vi "Simulated Console.vi"(8 "error in (no error)":errorcluster, 9 "Module Routes":refnum<user-event>[](array[refnum]), 11 "Event Registration Refnum":refnum<event-registration>) -> (0 "error out":errorcluster)   [LabVIEW 2018]
doc: "Simulated console UI"
uses:
  Architecture/Message Queue/Message Cluster.ctl
  Controls/Console Status.ctl
  Controls/Entry Display.ctl
  Car Wash Controller/Controls/Steps.ctl
  Car Wash Controller/Controls/Stations.ctl
  Architecture/Modules.ctl
  Controls/Button state.ctl
  Architecture/Message Queue/Message Queue.lvlib
panel:
  in  "Vehicle Position Simulation":u32(slide) scale=0.0..4.0
  out "Time Remaining":dbl format="%6.2f Seconds"
  out "Out of Position?":bool caption="Vehicle out of position"
  out "Air Dry":bool
  out "Tire Shine Foam":bool
  out "Spot Free Rinse":bool
  out "Low Pressure Wax":bool
  out "High Pressure Wash":bool
  out "Pre-Soak":bool
  out "Bug Remover":bool
  out "Under Body Wash":bool
  out "Wash Entry":string
  in  "Wash Start":bool
  in  "Air Dry":bool
  in  "Tire Shine Foam":bool
  in  "Spot Free Rinse":bool
  in  "Low Pressure Wax":bool
  in  "High Pressure Wash (default)":bool
  in  "Pre-Soak":bool
  in  "Bug Remover":bool
  in  "Under Body Wash":bool
  in  "debug":bool
  # "[Covers: UI2]\n[Covers UI2A]"
  # "[Covers: UI3]\n[Covers: UI3A]"
  # "[Covers: UI1]"
  # "Entry Console"
  # "Wash Display Console"
  # "[Covers: UI3B]\n[Covers: UI3B1]"
  # "[Covers: UI2B]"
  # "[Covers: UI3C]\n[Covers: UI3C1]\n[Covers: UI3C2]"
  # "[Covers: UI3D]\n[Covers: UI3D1]"
  # "Vehicle Position Simulation"
  # "[Covers: UI4]\n[Covers: UI4A]"
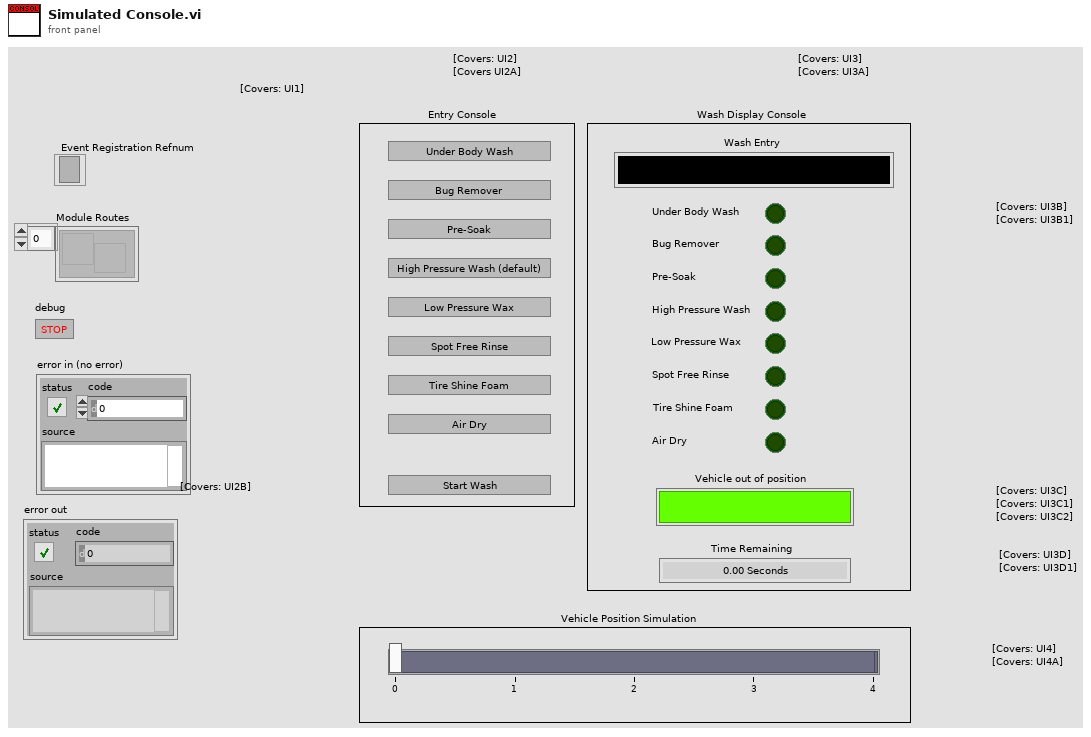
[diagram p1: front panel]
types:
  T1 = typedef "Console Status.ctl" = cluster{"Module Routes":refnum<user-event>[], "Chosen Cycles":cluster{"Under Body Wash":bool, "Bug Remover":bool, "Pre-Soak":bool, "High Pressure Wash (default)":bool, "Low Pressure Wax":bool, "Spot Free Rinse":bool, "Tire Shine Foam":bool, "Air Dry":bool}, "Entry Display":T2, "Current State":T3, "In Progress?":bool, "Out of Position?":bool, "Time Remaining":dbl, "Current Station":T4}
  T2 = typedef "Entry Display.ctl" = cluster{"Text":string, "Color":u32}
  T3 = typedef "Steps.ctl" = enum16{"Under Body Wash", "Bug Remover", "Pre-Soak", "High Pressure Wash", "Low Pressure Wax", "Spot Free Rinse", "Tire Shine Foam", "Air Dry"}
  T4 = typedef "Stations.ctl" = enum16{"Entry", "Station 1", "Station 2", "Station 3", "Exit"}
  T5 = typedef "Modules.ctl" = enum16{"Database", "Car Wash Controller", "Console"}
  T6 = typedef "Button state.ctl" = cluster{"Disabled State":enum8{"Enabled", "Disabled", "Disabled and Grayed Out"}, "State":bool}
  T7 = cluster{"[0]":bool, "[1]":bool, "[2]":bool, "[3]":bool, "[4]":bool, "[5]":bool, "[6]":bool, "[7]":bool}
  T8 = typedef "Error Severity.ctl" = enum16{"System Error", "Wash Error", "Minor"}
  T9 = cluster{"Under Body Wash":bool, "Bug Remover":bool, "Pre-Soak":bool, "High Pressure Wash (default)":bool, "Low Pressure Wax":bool, "Spot Free Rinse":bool, "Tire Shine Foam":bool, "Air Dry":bool}
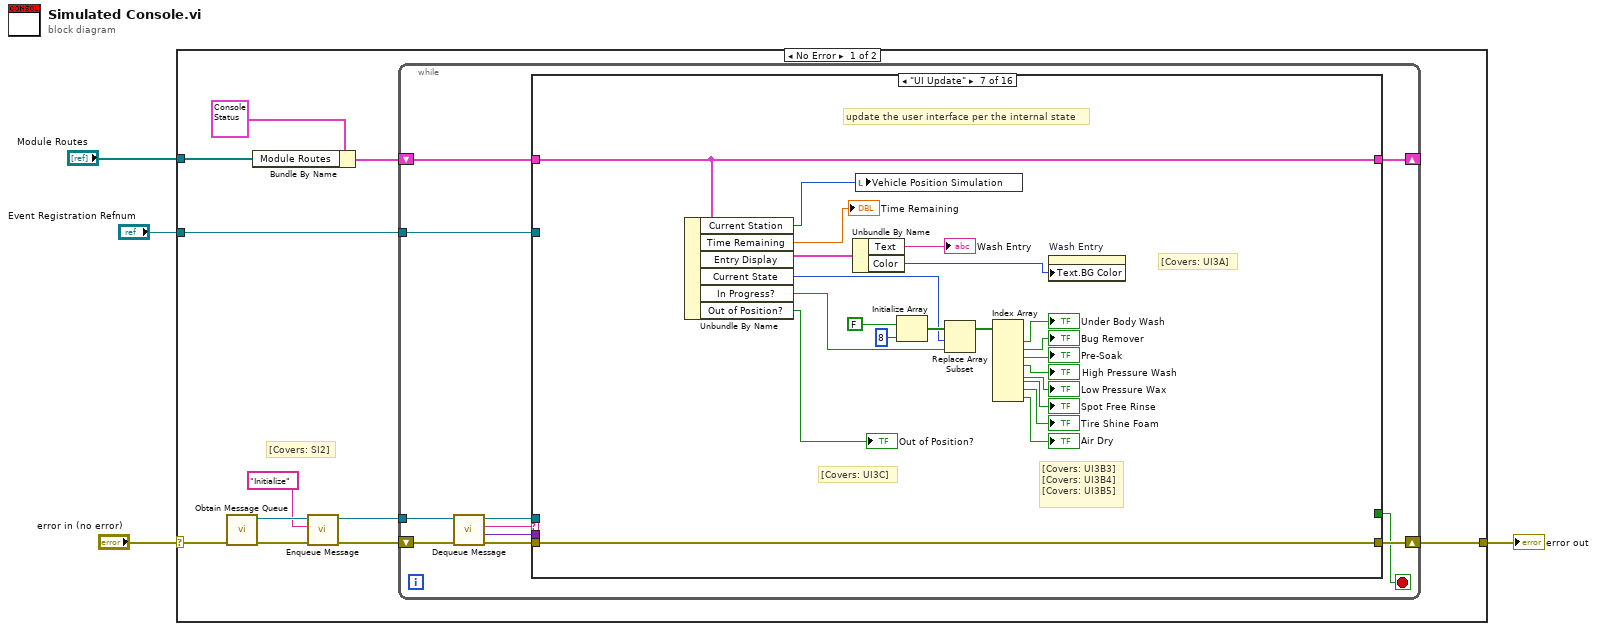
[diagram p0: block diagram]
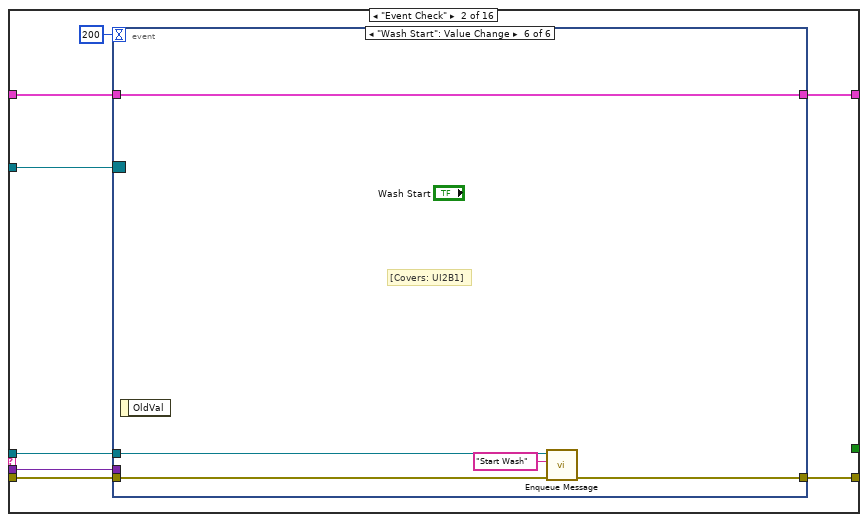
[diagram p3: hidden frame]
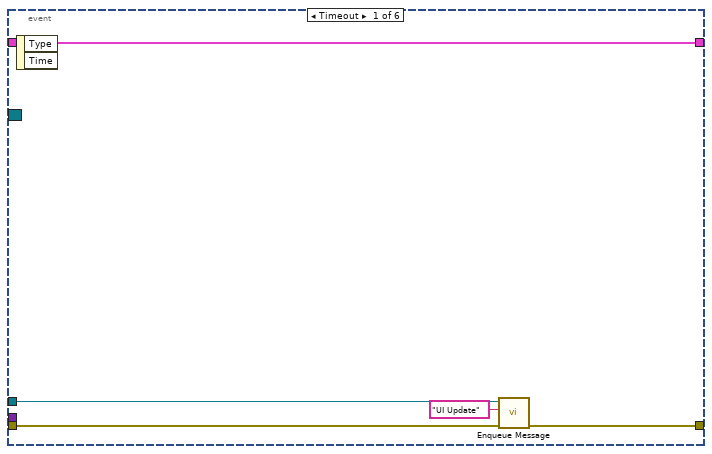
[diagram p4: hidden frame]
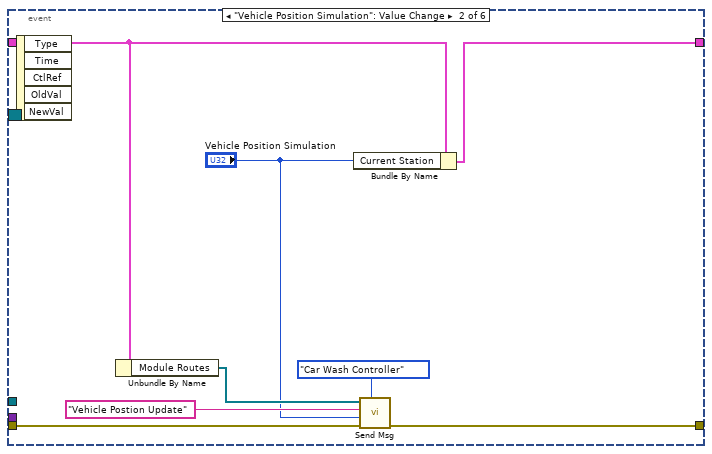
[diagram p5: hidden frame]
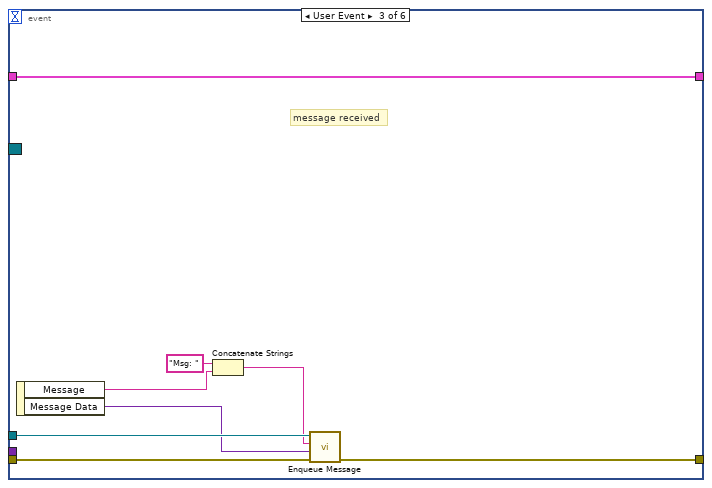
[diagram p6: hidden frame]
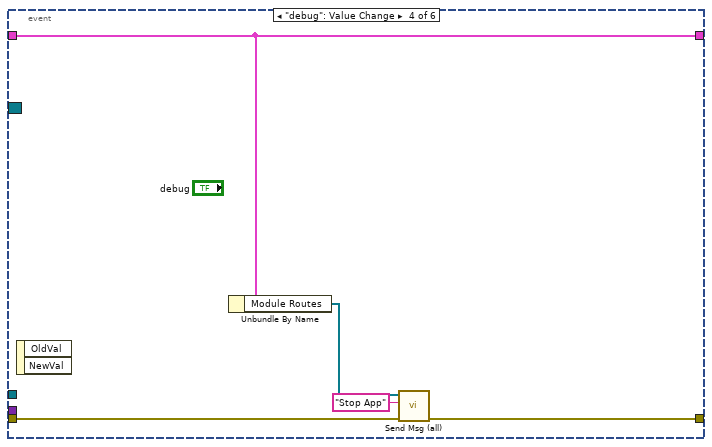
[diagram p7: hidden frame]
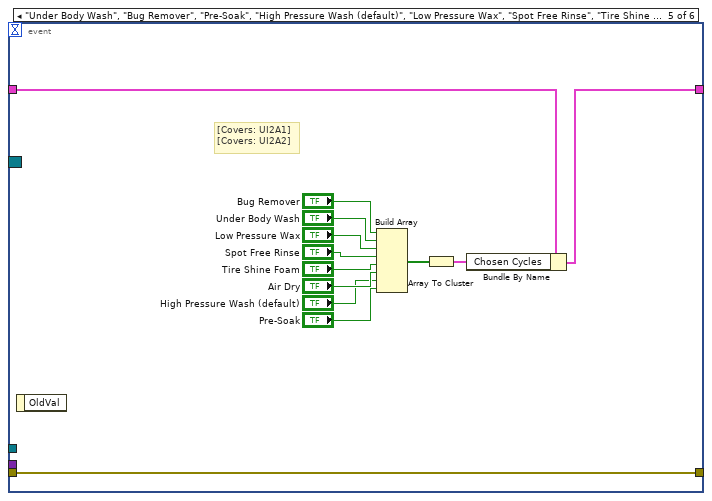
[diagram p8: hidden frame]
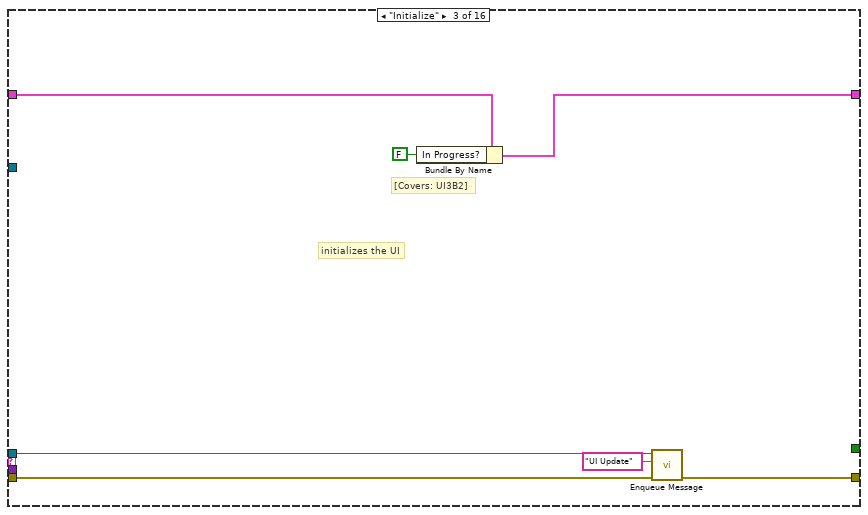
[diagram p9: hidden frame]
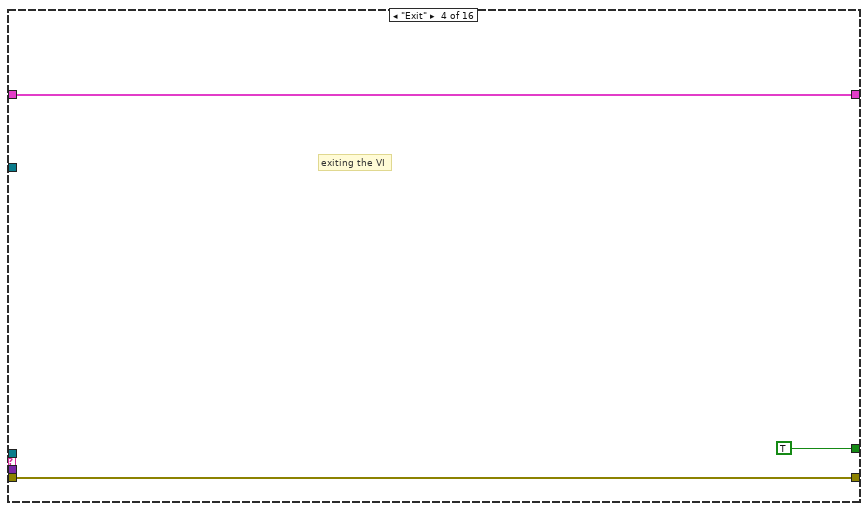
[diagram p10: hidden frame]
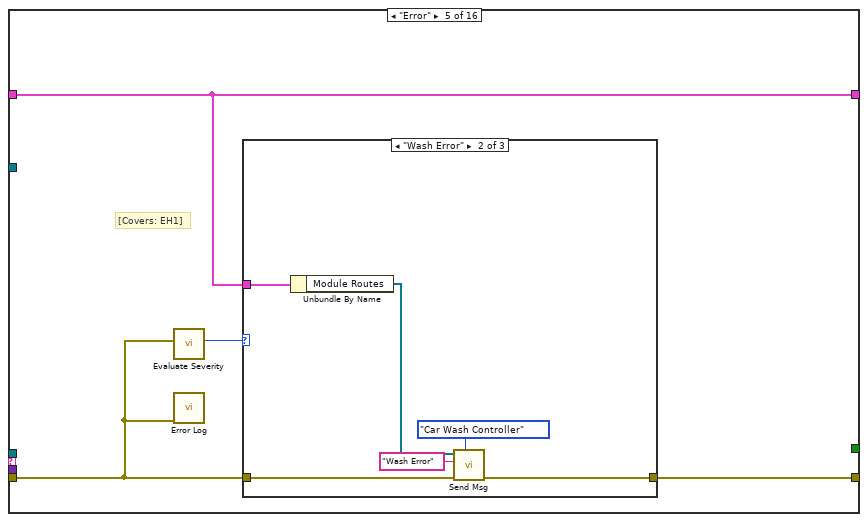
[diagram p11: hidden frame]
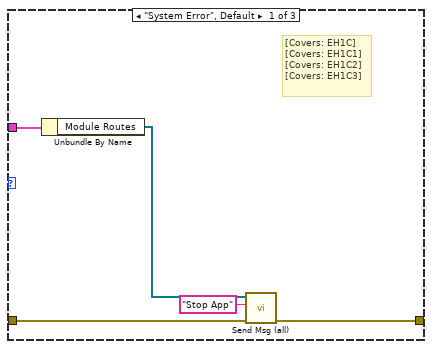
[diagram p12: hidden frame]
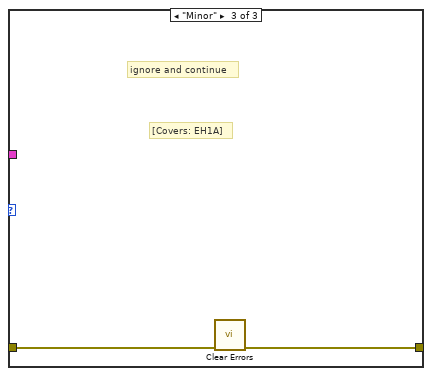
[diagram p13: hidden frame]
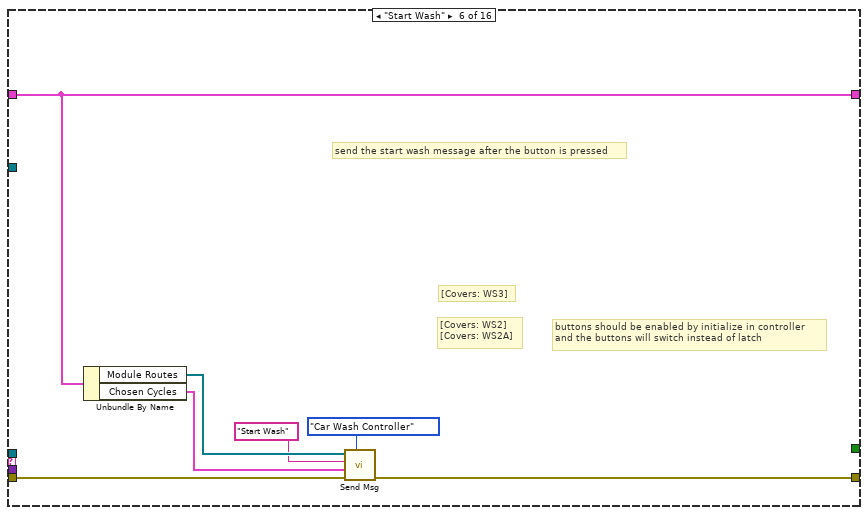
[diagram p14: hidden frame]
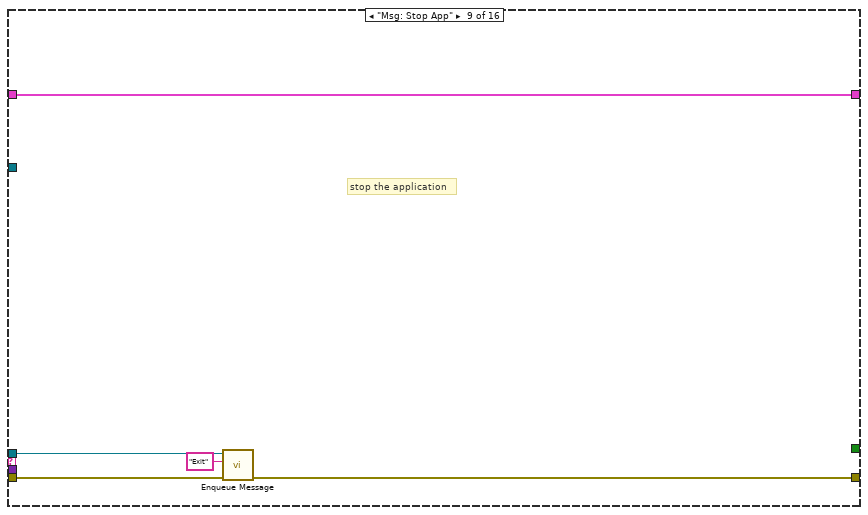
[diagram p16: hidden frame]
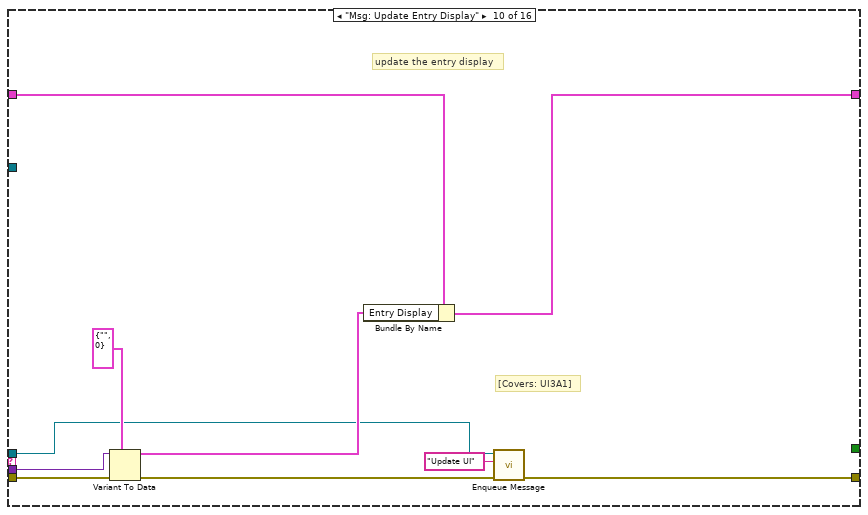
[diagram p17: hidden frame]
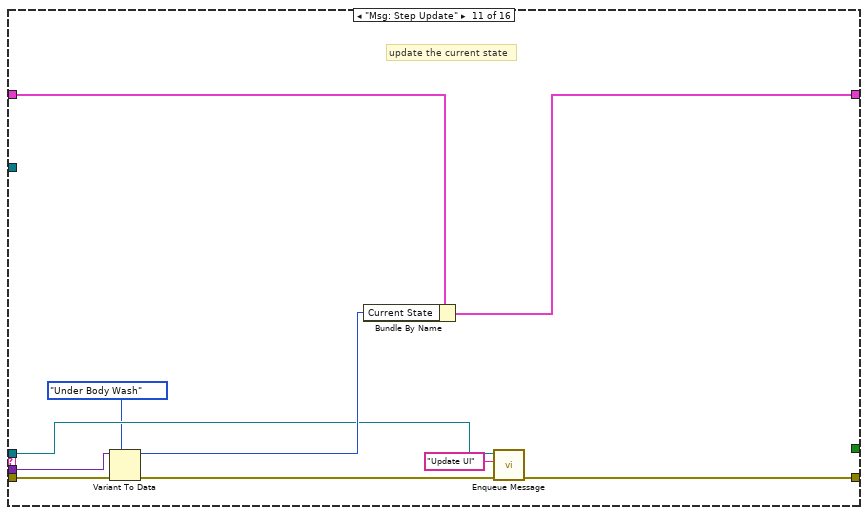
[diagram p18: hidden frame]
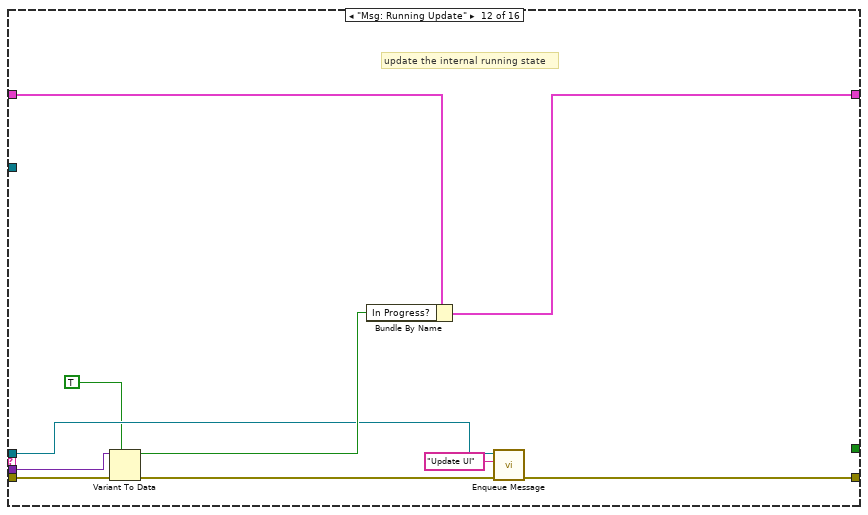
[diagram p19: hidden frame]
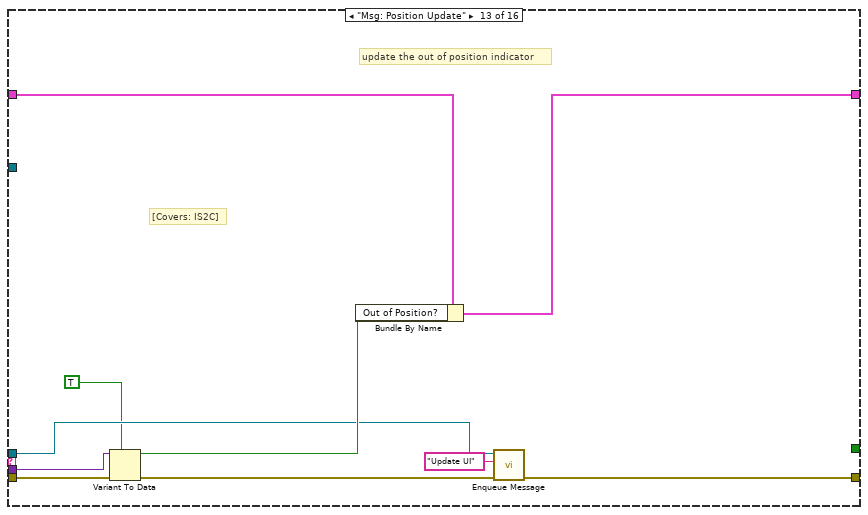
[diagram p20: hidden frame]
diagram:
  n1 = case shown="No Error" "error in (no error)" {
    selector: "error in (no error)" -> [w12 w220]
    tunnel: "Module Routes" -> [w14 _]
    tunnel: "Event Registration Refnum" -> [w13 _]
    tunnel: [w6 w220] -> w1
    frame No Error {
      # "[Covers: SI2]"
      n2 = call "Obtain Message Queue.vi"("error in (no error)"=w12) -> ("error out"=w11:errorcluster, "Message Queue"=w10:refnum<queue>)  [unwired: 9 in]
      n3 = Bundle By Name(cluster=T1 {"Module Routes"=[], "Chosen Cycles"={"Under Body Wash"=FALSE, "Bug Remover"=FALSE, "Pre-Soak"=FALSE, "High Pressure Wash (default)"=FALSE, "Low Pressure Wax"=FALSE, "Spot Free Rinse"=FALSE, "Tire Shine Foam"=FALSE, "Air Dry"=FALSE}, "Entry Display"={"Text"="", "Color"=0}, "Current State"=enum."Under Body Wash", "In Progress?"=FALSE, "Out of Position?"=FALSE, "Time Remaining"=0.0, "Current Station"=enum."Entry"} ("Status"), "Module Routes"=w14) -> (w5:T1)
      n4 = call "Enqueue Message.vi"("error in (no error)"=w11, "Message"="Initialize", "Message Queue"=w10) -> ("error out"=w8:errorcluster, "dup Message Queue"=w7:refnum<queue>)  [unwired: 7 in]
      n5 = while {
        tunnel: w13 -> [w26]
        shift-right: [w22] -> w6
        shift-left: w8 -> [w25]
        tunnel: w7 -> [w24]
        shift-right: [w16] -> _
        shift-left: w5 -> [w17]
        stop <- w18 stop-if-true
        n6 = call "Dequeue Message.vi"("error in (no error)"=w25, "Message Queue"=w24) -> ("error out"=w23:errorcluster, "Message Data"=w20:variant, "Message"=w19:string, "dup Message Queue"=w21:refnum<queue>)  [unwired: 6 in]
        n7 = case shown="\"UI Update\"" w19 {
          tunnel: w26 -> [_ w36 _ _ _ _ _ _ _ _ _ _ _ _ _ _]
          tunnel: w23 -> [w28 w35 w84 w90 w91 w114 w136 w138 w142 w153 w163 w173 w183 w193 w203 w219]
          tunnel: [w28 w34 w82 w90 w93 w113 w136 w138 w140 w144 w155 w165 w175 w185 w196 w216] -> w22
          tunnel: w21 -> [_ w33 w83 _ _ _ _ _ w141 w146 w157 w167 w177 w187 w198 _]
          tunnel: w20 -> [_ w32 _ _ _ _ _ _ _ w151 w162 w172 w182 w192 w202 w218]
          tunnel: [_ _ _ TRUE _ _ _ _ _ _ _ _ _ _ _ _] -> w18
          tunnel: w17 -> [w27 w31 w87 w88 w92 w112 w135 w137 w143 w150 w161 w171 w181 w191 w201 w215]
          tunnel: [w27 w30 w86 w88 w92 w112 w135 w137 w143 w149 w160 w170 w180 w190 w200 w215] -> w16
          frame Default {
            # "invalid case"
          }
          frame "Event Check" {
            n8 = event shown="[5] \"Wash Start\": Value Change" {
              selector: w36 -> [_ _ _ _ _ _]
              dyn-events: _ -> [_ _ _ _ _ _]
              timeout: 200 -> [_ _ _ _ _ _]
              tunnel: [w39 w47 w54 w61 w75 w78] -> w34
              tunnel: w35 -> [w40 w48 w55 w62 w75 w79]
              tunnel: w33 -> [w38 _ w53 _ _ w77]
              tunnel: w32 -> [_ _ _ _ _ _]
              tunnel: w31 -> [w41 w45 w50 w60 w65 w80]
              tunnel: [w41 w49 w50 w60 w64 w80] -> w30
              event Timeout {
                n9 = event-data() -> ()  [unwired: 1 in, 2 out]
                n10 = call "Enqueue Message.vi"("error in (no error)"=w40, "Message"="UI Update", "Message Queue"=w38) -> ("error out"=w39:errorcluster)  [unwired: 7 in, 1 out]
              }
              event "Vehicle Position Simulation": Value Change {
                n11 = event-data() -> ()  [unwired: 1 in, 5 out]
                n12 = Unbundle By Name(w45) -> ("Module Routes"=w44:refnum<user-event>[])
                n13 = Bundle By Name(cluster=w45, "Current Station"="Vehicle Position Simulation") -> (w49:T1)
                n14 = call "Send Msg.vi"("Module"=Modules."Car Wash Controller", "error in (no error)"=w48, "Message Data"="Vehicle Position Simulation", "Message"="Vehicle Postion Update", "Module Routes"=w44) -> ("error out"=w47:errorcluster)  [unwired: 6 in]
              }
              event User Event {
                # "message received"
                n15 = event-data() -> ("Message"=w56:string, "Message Data"=w52:variant)  [unwired: 1 in]
                n16 = Concatenate Strings("Msg: " ("string"), w56) -> (w51:string)
                n17 = call "Enqueue Message.vi"("error in (no error)"=w55, "Message Data"=w52, "Message"=w51, "Message Queue"=w53) -> ("error out"=w54:errorcluster)  [unwired: 6 in, 1 out]
              }
              event "debug": Value Change {
                n18 = event-data() -> ()  [unwired: 1 in, 2 out]
                n19 = Unbundle By Name(w60) -> ("Module Routes"=w59:refnum<user-event>[])
                n20 = call "Send Msg (all).vi"("error in (no error)"=w62, "Message"="Stop App", "Module Routes"=w59) -> ("error out"=w61:errorcluster)  [unwired: 8 in]
              }
              event "Under Body Wash", "Bug Remover", "Pre-Soak", "High Pressure Wash (default)", "Low Pressure Wax", "Spot Free Rinse", "Tire Shine Foam", "Air Dry": Value Change {
                # "[Covers: UI2A1]\n[Covers: UI2A2]"
                n21 = event-data() -> ()  [unwired: 1 in, 1 out]
                n22 = Build Array("Bug Remover", "Under Body Wash", "Low Pressure Wax", "Spot Free Rinse", "Tire Shine Foam", "Air Dry", "High Pressure Wash (default)", "Pre-Soak") -> (w66:bool[])
                n23 = Array To Cluster(array=w66) -> (cluster=w63:T7)
                n24 = Bundle By Name(cluster=w65, "Chosen Cycles"=w63) -> (w64:T1)
              }
              event "Wash Start": Value Change {
                # "[Covers: UI2B1]"
                n25 = event-data() -> ()  [unwired: 1 in, 1 out]
                n26 = call "Enqueue Message.vi"("error in (no error)"=w79, "Message"="Start Wash", "Message Queue"=w77) -> ("error out"=w78:errorcluster)  [unwired: 7 in, 1 out]
              }
            }
          }
          frame "Initialize" {
            # "initializes the UI"
            # "[Covers: UI3B2]"
            n27 = Bundle By Name(cluster=w87, "In Progress?"=FALSE) -> (w86:T1)
            n28 = call "Enqueue Message.vi"("error in (no error)"=w84, "Message"="UI Update", "Message Queue"=w83) -> ("error out"=w82:errorcluster)  [unwired: 7 in, 1 out]
          }
          frame "Exit" {
            # "exiting the VI"
          }
          frame "Error" {
            # "[Covers: EH1]"
            n29 = call "Evaluate Severity.vi"("error in (no error)"=w91) -> ("Severity"=w94:T8)  [unwired: 10 in]
            n30 = call "Error Log.vi"("error in (no error)"=w91) -> ()  [unwired: 11 in]
            n31 = case shown="\"Wash Error\"" w94 {
              tunnel: w91 -> [w99 w104 w107]
              tunnel: [w98 w105 w106] -> w93
              tunnel: w92 -> [w97 w103 _]
              frame "System Error", Default {
                # "[Covers: EH1C]\n[Covers: EH1C1]\n[Covers: EH1C2]\n[Covers: EH1C3]"
                n32 = Unbundle By Name(w97) -> ("Module Routes"=w96:refnum<user-event>[])
                n33 = call "Send Msg (all).vi"("error in (no error)"=w99, "Message"="Stop App", "Module Routes"=w96) -> ("error out"=w98:errorcluster)  [unwired: 8 in]
              }
              frame "Wash Error" {
                n34 = Unbundle By Name(w103) -> ("Module Routes"=w102:refnum<user-event>[])
                n35 = call "Send Msg.vi"("Module"=Modules."Car Wash Controller", "error in (no error)"=w104, "Message"="Wash Error", "Module Routes"=w102) -> ("error out"=w105:errorcluster)  [unwired: 7 in]
              }
              frame "Minor" {
                # "[Covers: EH1A]"
                # "ignore and continue"
                n36 = call <vilib>:"Clear Errors.vi"("error in (no error)"=w107) -> ("error out"=w106:errorcluster)  [unwired: 5 in, 1 out]
              }
            }
          }
          frame "Start Wash" {
            # "send the start wash message after the button is pressed"
            # "buttons should be enabled by initialize in controller\nand the buttons will switch instead of latch"
            # "[Covers: WS2]\n[Covers: WS2A]"
            # "[Covers: WS3]"
            n37 = Unbundle By Name(w112) -> ("Module Routes"=w110:refnum<user-event>[], "Chosen Cycles"=w108:T9)
            n38 = call "Send Msg.vi"("Module"=Modules."Car Wash Controller", "error in (no error)"=w114, "Message Data"=w108, "Message"="Start Wash", "Module Routes"=w110) -> ("error out"=w113:errorcluster)  [unwired: 6 in]
          }
          frame "UI Update" {
            # "update the user interface per the internal state"
            # "[Covers: UI3A]"
            # "[Covers: UI3C]"
            # "[Covers: UI3B3]\n[Covers: UI3B4]\n[Covers: UI3B5]"
            n39 = Unbundle By Name(w135) -> ("Current Station"=w115:T4, "Time Remaining"=→"Time Remaining":dbl, "Entry Display"=w134:T2, "Current State"=w119:T3, "In Progress?"=w118:bool, "Out of Position?"=→"Out of Position?":bool)
            n40 = Unbundle By Name(w134) -> ("Text"=→"Wash Entry":string, "Color"=w132:u32)
            n41 = local write "Vehicle Position Simulation"(w115) -> ()
            n42 = Initialize Array(FALSE, 8 ("dimension size")) -> (w121:bool[])
            n43 = Replace Array Subset(array=w121, new element=w118, index=w119) -> (w120:bool[])
            n44 = Index Array(array=w120) -> (element #1=→"Under Body Wash":bool, element #2=→"Bug Remover":bool, element #3=→"Pre-Soak":bool, element #4=→"High Pressure Wash":bool, element #5=→"Low Pressure Wax":bool, element #6=→"Spot Free Rinse":bool, element #7=→"Tire Shine Foam":bool, element #8=→"Air Dry":bool)  [unwired: 8 in]
            n45 = property on="Wash Entry" class="Str"("Text.BG Color"=w132) -> ()  [unwired: 2 in, 2 out]
          }
          frame "=== Messages ===" {
            # "placeholder"
          }
          frame "Msg: Stop App" {
            # "stop the application"
            n46 = call "Enqueue Message.vi"("error in (no error)"=w142, "Message"="Exit", "Message Queue"=w141) -> ("error out"=w140:errorcluster)  [unwired: 7 in, 1 out]
          }
          frame "Msg: Update Entry Display" {
            # "update the entry display"
            # "[Covers: UI3A1]"
            n47 = Variant To Data(error in=w153, type=T2 {"Text"="", "Color"=0}, Variant=w151) -> (data=w148:T2, error out=w147:errorcluster)
            n48 = Bundle By Name(cluster=w150, "Entry Display"=w148) -> (w149:T1)
            n49 = call "Enqueue Message.vi"("error in (no error)"=w147, "Message"="Update UI", "Message Queue"=w146) -> ("error out"=w144:errorcluster)  [unwired: 7 in, 1 out]
          }
          frame "Msg: Step Update" {
            # "update the current state"
            n50 = Variant To Data(error in=w163, type=Steps."Under Body Wash" ("Current State"), Variant=w162) -> (data=w159:T3, error out=w158:errorcluster)
            n51 = Bundle By Name(cluster=w161, "Current State"=w159) -> (w160:T1)
            n52 = call "Enqueue Message.vi"("error in (no error)"=w158, "Message"="Update UI", "Message Queue"=w157) -> ("error out"=w155:errorcluster)  [unwired: 7 in, 1 out]
          }
          frame "Msg: Running Update" {
            # "update the internal running state"
            n53 = Variant To Data(error in=w173, type=TRUE, Variant=w172) -> (data=w169:bool, error out=w168:errorcluster)
            n54 = Bundle By Name(cluster=w171, "In Progress?"=w169) -> (w170:T1)
            n55 = call "Enqueue Message.vi"("error in (no error)"=w168, "Message"="Update UI", "Message Queue"=w167) -> ("error out"=w165:errorcluster)  [unwired: 7 in, 1 out]
          }
          frame "Msg: Position Update" {
            # "update the out of position indicator"
            # "[Covers: IS2C]"
            n56 = Variant To Data(error in=w183, type=TRUE, Variant=w182) -> (data=w179:bool, error out=w178:errorcluster)
            n57 = Bundle By Name(cluster=w181, "Out of Position?"=w179) -> (w180:T1)
            n58 = call "Enqueue Message.vi"("error in (no error)"=w178, "Message"="Update UI", "Message Queue"=w177) -> ("error out"=w175:errorcluster)  [unwired: 7 in, 1 out]
          }
          frame "Msg: Station Update" {
            # "update the current station"
            # "[Covers: IS3]"
            n59 = Variant To Data(error in=w193, type=Stations."Entry" ("Stations"), Variant=w192) -> (data=w189:T4, error out=w188:errorcluster)
            n60 = Bundle By Name(cluster=w191, "Current Station"=w189) -> (w190:T1)
            n61 = call "Enqueue Message.vi"("error in (no error)"=w188, "Message"="Update UI", "Message Queue"=w187) -> ("error out"=w185:errorcluster)  [unwired: 7 in, 1 out]
          }
          frame "Msg: Timing Update" {
            # "update the time remaining"
            # "[Covers: IS2D]"
            n62 = Variant To Data(error in=w203, type=0.0, Variant=w202) -> (data=w194:dbl, error out=w199:errorcluster)
            n63 = Bundle By Name(cluster=w201, "Time Remaining"=w194) -> (w200:T1)
            n64 = call "Enqueue Message.vi"("error in (no error)"=w199, "Message"="Update UI", "Message Queue"=w198) -> ("error out"=w196:errorcluster)  [unwired: 7 in, 1 out]
          }
          frame "Msg: Button States" {
            # "update the state of the buttons (enabled/disabled)"
            # "[Covers: UI2A3]\n[Covers: UI2A4]"
            # "[Covers: IS1]"
            # "This state will update the Entry Console buttons\nbased upon the message received.  The array is assumed\nto be in the order of the buttons on screen from \ntop to bottom."
            n65 = Variant To Data(error in=w219, type=T6[] [], Variant=w218) -> (data=w204:T6[], error out=w216:errorcluster)
            n66 = control-ref of="Under Body Wash"() -> (w206:refnum<vi>)
            n67 = control-ref of="Bug Remover"() -> (w207:refnum<vi>)
            n68 = control-ref of="Pre-Soak"() -> (w208:refnum<vi>)
            n69 = control-ref of="High Pressure Wash (default)"() -> (w209:refnum<vi>)
            n70 = control-ref of="Air Dry"() -> (w210:refnum<vi>)
            n71 = control-ref of="Tire Shine Foam"() -> (w211:refnum<vi>)
            n72 = control-ref of="Spot Free Rinse"() -> (w212:refnum<vi>)
            n73 = control-ref of="Low Pressure Wax"() -> (w213:refnum<vi>)
            n74 = control-ref of="Wash Start"() -> (w214:refnum<vi>)
            n75 = Build Array(w206, w207, w208, w209, w210, w211, w212, w213, w214) -> (w205:refnum<vi>[])
            n76 = call "Set Button States.vi"("Button States"=w204, "Button References"=w205) -> ()  [unwired: 10 in]
          }
        }
      }
    }
    frame Error {
    }
  }
  "error out" <- w1
